vi "convert_labview_signal_files_small.vi"(5 "Convert":bool, 7 "Keep file names?":bool=TRUE, 8 "error in":errorcluster, 10 "Save Path":path, 11 "Open Path":path=path "Z:/DatabaseProject/LV test") -> (0 "error out":errorcluster)   [LabVIEW 2013]
uses:
  Public API/Signal.ctl
  Private/Role ID.ctl
  Private/Hardware ID.ctl
panel:
  in  "Signal array":T1[](array[typedef])
  out "Slide":u8(slide) scale=0.0..100.0
  out "Number of files to be converted:":dbl
  in  "stop":bool
  # "CCLDAS File Conversion System"
  # "Signal"
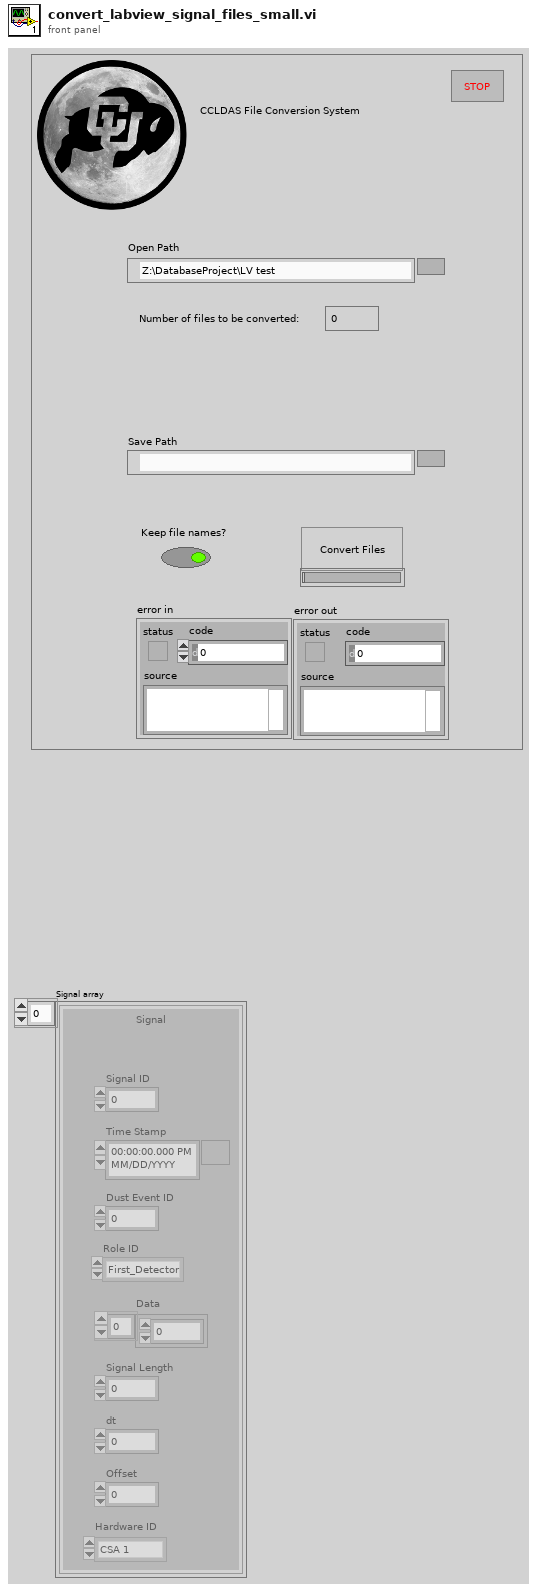
[diagram p1: front panel]
types:
  T1 = typedef "Signal.ctl" = cluster{"Signal ID":i64, "Time Stamp":timestamp, "Dust Event ID":i64, "Role ID":T2, "Data":sgl[], "Signal Length":i32, "dt":sgl, "Offset":dbl, "Hardware ID":T3}
  T2 = typedef "Role ID.ctl" = enum16{"First_Detector", "Second_Detector", "Third_Detector", "LeCroy_CH1", "LeCroy_CH2", "LeCroy_CH3", "LeCroy_CH4", "PSU"}
  T3 = typedef "Hardware ID.ctl" = enum16{"Unknown", "CSA 1", "CSA 2", "CSA 3", "CSA 4", "CSA 5", "CSA 6"}
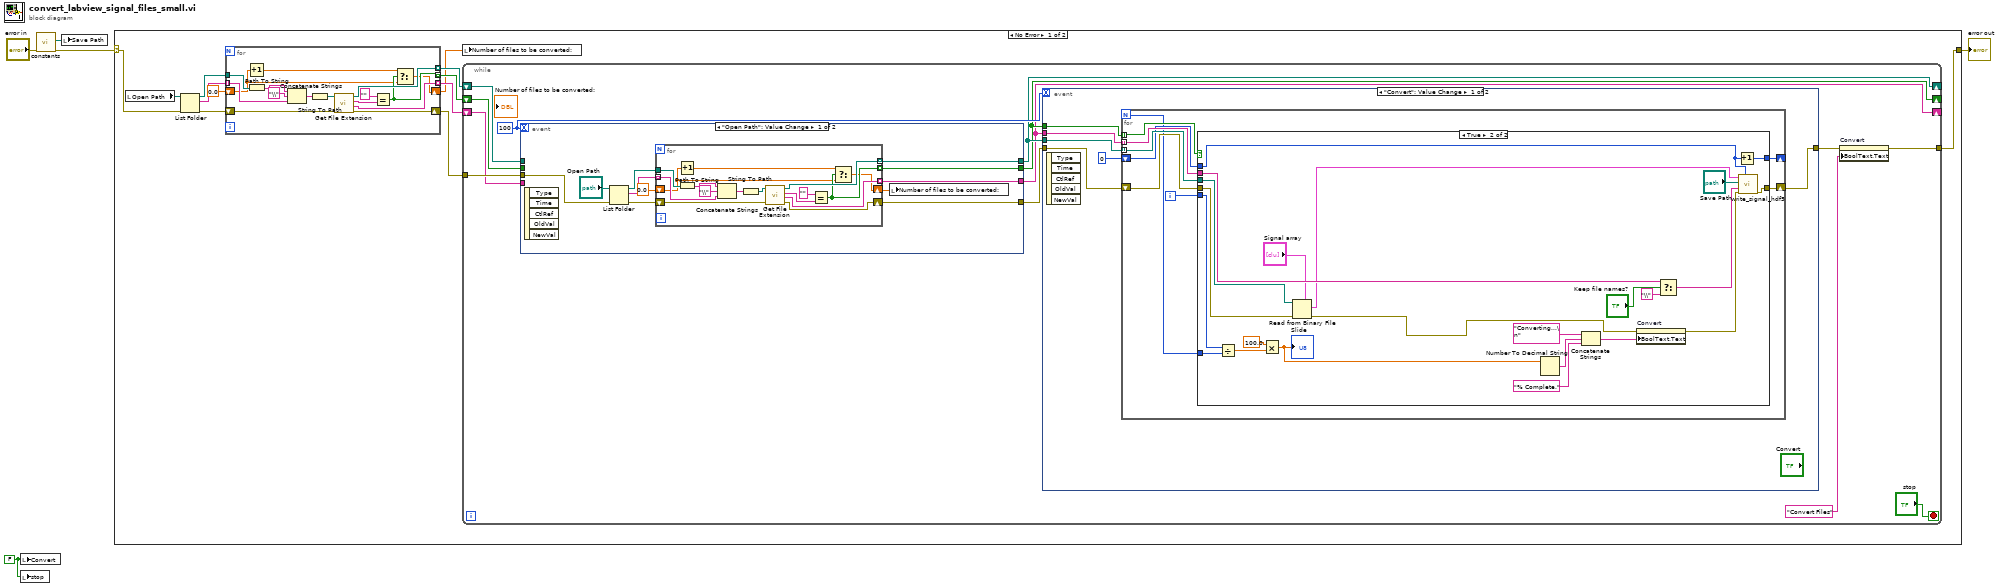
[diagram p0: block diagram]
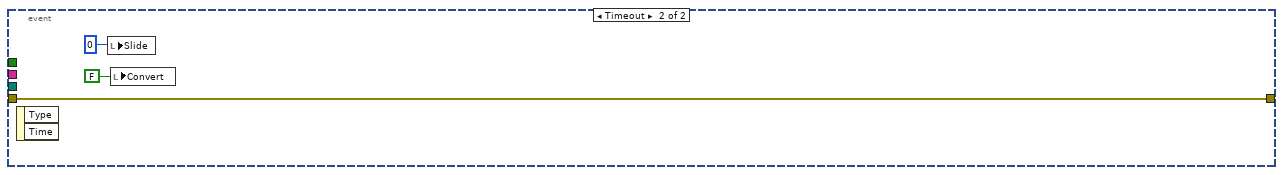
[diagram p3: hidden frame]
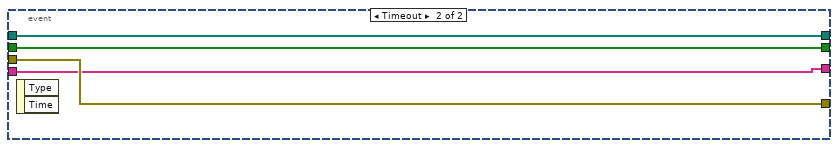
[diagram p4: hidden frame]
diagram:
  w4 = FALSE ("Convert")
  n1 = local write "Convert"(w4) -> ()
  n2 = local write "stop"(w4) -> ()
  n3 = call "constants.vi"("error in (no error)"="error in") -> ("error out"=w1:errorcluster, "file path for Signal .hdf5 files"=w3:path)  [unwired: 4 in, 5 out]
  n4 = local write "Save Path"(w3) -> ()
  n5 = case shown="No Error" w1 {
    selector: w1 -> [w11 w121]
    tunnel: [w17 w121] -> w5
    frame No Error {
      n6 = local read "Open Path"() -> (w12:path)
      n7 = List Folder(path=w12, error in=w11) -> (path out=w15:path, filenames=w16:string[], error out=w14:errorcluster)  [unwired: 2 in, 1 out]
      n8 = for {
        tunnel: w16 -> [w28] mode=indexing
        tunnel: w15 -> [w27]
        tunnel: [w25] -> w8 mode=indexing
        shift-right: [w23] -> w10
        shift-left: w14 -> [w24]
        tunnel: [w22] -> w7 mode=indexing
        tunnel: [w21] -> w9 mode=indexing
        shift-right: [w19] -> w6
        shift-left: 0.0 -> [w18]
        n9 = Increment(x=w18) -> (x+1=w20:dbl)
        n10 = Path To String(path=w27) -> (string=w30:string)
        n11 = Concatenate Strings(w30, "\\" ("x"), w28) -> (w31:string)
        n12 = String To Path(string=w31) -> (path=w26:path)
        n13 = call <vilib>:"Get File Extension.vi"("error in (no error)"=w24, "file"=w26) -> ("error out"=w23:errorcluster, "filename without extension"=w22:string, "lowercase file extension"=w32:string, "dup file"=w25:path)  [unwired: 6 in]
        n14 = Equal?(x="" ("lowercase file extension"), y=w32) -> (x = y?=w21:bool)
        n15 = Select(t=w20, s=w21, f=w18) -> (s? t:f=w19:dbl)
      }
      n16 = local write "Number of files to be converted:"(w6) -> ()
      n17 = while {
        tunnel: [w35] -> w17
        tunnel: w10 -> [w46]
        shift-right: [w42] -> _
        shift-left: w8 -> [w38]
        shift-right: [w41] -> _
        shift-left: w9 -> [w37]
        shift-right: [w40] -> _
        shift-left: w7 -> [w39]
        stop <- "stop" stop-if-true
        w44 = 100
        n18 = event shown="[0] \"Open Path\": Value Change" {
          selector: _ -> [_ _]
          dyn-events: _ -> [_ _]
          timeout: w44 -> [_ _]
          tunnel: w46 -> [w100 w120]
          tunnel: [w96 w118] -> w42
          tunnel: [w94 w120] -> w45
          tunnel: [w93 w119] -> w40
          tunnel: [w92 w117] -> w41
          tunnel: w39 -> [_ w119]
          tunnel: w38 -> [_ w118]
          tunnel: w37 -> [_ w117]
          event "Open Path": Value Change {
            n19 = event-data() -> ()  [unwired: 1 in, 5 out]
            n20 = List Folder(path="Open Path", error in=w100) -> (path out=w97:path, filenames=w98:string[], error out=w95:errorcluster)  [unwired: 2 in, 1 out]
            n21 = for {
              tunnel: w98 -> [w111] mode=indexing
              tunnel: w97 -> [w110]
              tunnel: [w108] -> w96 mode=indexing
              shift-right: [w106] -> w94
              shift-left: w95 -> [w107]
              tunnel: [w105] -> w93 mode=indexing
              tunnel: [w104] -> w92 mode=indexing
              shift-right: [w102] -> w90
              shift-left: 0.0 -> [w101]
              n22 = Increment(x=w101) -> (x+1=w103:dbl)
              n23 = Path To String(path=w110) -> (string=w113:string)
              n24 = Concatenate Strings(w113, "\\" ("x"), w111) -> (w114:string)
              n25 = String To Path(string=w114) -> (path=w109:path)
              n26 = call <vilib>:"Get File Extension.vi"("error in (no error)"=w107, "file"=w109) -> ("error out"=w106:errorcluster, "filename without extension"=w105:string, "lowercase file extension"=w115:string, "dup file"=w108:path)  [unwired: 6 in]
              n27 = Equal?(x="" ("lowercase file extension"), y=w115) -> (x = y?=w104:bool)
              n28 = Select(t=w103, s=w104, f=w101) -> (s? t:f=w102:dbl)
            }
            n29 = local write "Number of files to be converted:"(w90) -> ()
          }
          event Timeout {
            n30 = event-data() -> ()  [unwired: 1 in, 2 out]
          }
        }
        n31 = event shown="[0] \"Convert\": Value Change" {
          selector: _ -> [_ _]
          dyn-events: _ -> [_ _]
          timeout: w44 -> [_ _]
          tunnel: [w52 w89] -> w36
          tunnel: w42 -> [w51 _]
          tunnel: w45 -> [w50 w89]
          tunnel: w40 -> [w49 _]
          tunnel: w41 -> [w48 _]
          event "Convert": Value Change {
            n32 = event-data() -> ()  [unwired: 1 in, 5 out]
            n33 = for {
              N -> [w53]
              shift-right: [w61] -> w52
              shift-left: w50 -> [w58]
              tunnel: w51 -> [w60] mode=indexing
              tunnel: w49 -> [w59] mode=indexing
              tunnel: w48 -> [w57] mode=indexing
              shift-right: [w55] -> _
              shift-left: 0 ("Offset") -> [w56]
              i -> [w54]
              n34 = case shown="True" w57 {
                tunnel: [w63 w86] -> w61
                tunnel: w60 -> [_ w67]
                tunnel: w59 -> [_ w81]
                tunnel: w58 -> [w63 w66]
                tunnel: w56 -> [w62 w80]
                tunnel: [w62 w79] -> w55
                tunnel: w54 -> [_ w78]
                tunnel: w53 -> [_ w69]
                frame False {
                }
                frame True {
                  n35 = Divide(x=w78, y=w69) -> (x/y=w77:dbl)
                  n36 = Multiply(x=100.0, y=w77) -> (x*y=w70:dbl)
                  "Slide" <- w70
                  n37 = Read from Binary File(5:"Signal array", 8:w66, 11:w67) -> (0:w68:errorcluster, 2:w64:T1[])  [unwired: 3 in, 2 out]
                  n38 = Number To Decimal String(number=w70) -> (decimal integer string=w74:string)  [unwired: 1 in]
                  n39 = Concatenate Strings("Converting...\n" ("string"), w74, "% Complete." ("string")) -> (w71:string)
                  n40 = property on="Convert" class="Bool (strict)"(error in=w68, "BoolText.Text"=w71) -> (error out=w75:errorcluster)  [unwired: 1 in, 1 out]
                  n41 = Select(t=w81, s="Keep file names?", f="\\") -> (s? t:f=w82:string)
                  n42 = Increment(x=w80) -> (x+1=w79:i32)
                  n43 = call "write_signal_hdf5.vi"("Index"=w80, "error in"=w75, "File Name"=w82, "Save Path"="Save Path", "Signal array"=w64) -> ("error out"=w86:errorcluster)  [unwired: 5 in, 1 out]
                }
              }
            }
          }
          event Timeout {
            n44 = event-data() -> ()  [unwired: 1 in, 2 out]
            n45 = local write "Slide"(u8 0 ("Slide")) -> ()
            n46 = local write "Convert"(FALSE ("Convert")) -> ()
          }
        }
        n47 = property on="Convert" class="Bool (strict)"(error in=w36, "BoolText.Text"="Convert Files" ("Boolean Text.Text")) -> (error out=w35:errorcluster)  [unwired: 1 in, 1 out]
      }
    }
    frame Error {
    }
  }
  "error out" <- w5
